vi "Autonomous Independent.vi"() -> ()   [LabVIEW 2014]
doc: "This VI is called when autonomous begins, and will automatically be terminated when autonomous ends. You can carry out timed or sensor driven robot movement independently without needing to return to the caller."
uses:
  Robot Global Data.vi
  <vilib>/Rock Robotics/WPI/RobotDrive/WPI_RobotDriveGetSetRefNum.vi
  <vilib>/Rock Robotics/WPI/RobotDrive/WPI_RobotDriveMecanumDrive_Cartesian.vi
panel:
  out "Current Movement, for debugging":T1 {"Z Joystick Value" scale=-1.0..1.0; "Y Joystick Value" scale=1.0..-1.0; "X Joystick Value" scale=-1.0..1.0}
  in  "Array of robot movements":T2(array[cluster]) {"Z Joystick Value" scale=-1.0..1.0; "Y Joystick Value" scale=1.0..-1.0; "X Joystick Value" scale=-1.0..1.0}
  # "Be sure to right-click and choose Data Operations>>Make Current Value default if you want to save the array values with the VI"
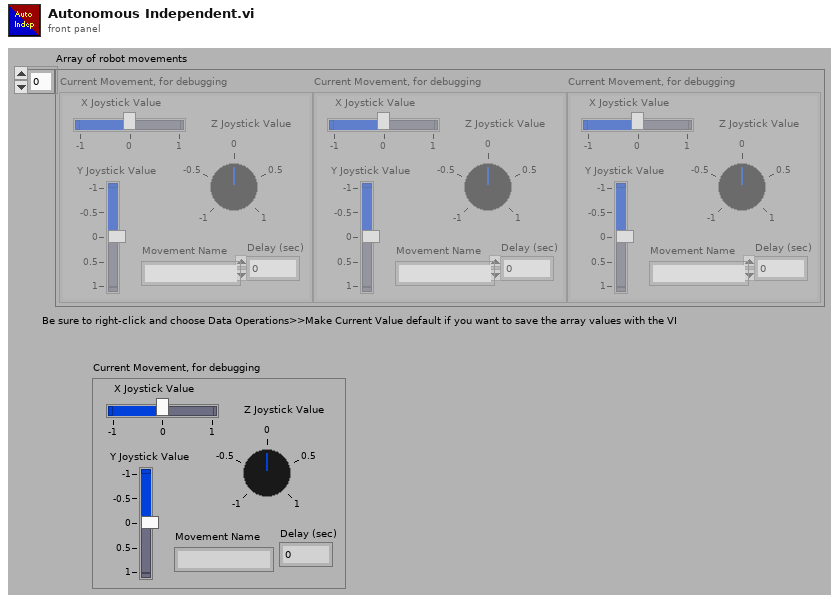
[diagram p1: front panel]
types:
  T1 = cluster{"X Joystick Value":dbl, "Y Joystick Value":dbl, "Z Joystick Value":dbl, "Delay (sec)":dbl, "Movement Name":string}
  T2 = cluster{"X Joystick Value":dbl, "Y Joystick Value":dbl, "Z Joystick Value":dbl, "Delay (sec)":dbl, "Movement Name":string}[]
  T3 = typedef "WPI_RobotDriveDevRef.ctl" = cluster{"DevStatus":errorcluster, "Motors[]":T4[], "Square Inputs":bool, "Max Output":dbl}
  T4 = typedef "WPI_MotorControlDeviceRef.ctl" = cluster{"DeviceStatus":errorcluster, "Type":enum16{"PWM", "CAN"}, "PWM":cluster{"Digital Module":T5, "PWM Channel":T6, "DeadBand":T7}, "CAN":cluster{"Device Number":u8, "Control Mode":T8, "Semaphore":T9, "Max Vout":dbl}, "Invert":bool, "TransformRef":T10, "InvTransformRef":T10}
  T5 = typedef "FPGA_TypedefDigitalModule.ctl" = enum16{"Digital Module 1", "Digital Module 2"}
  T6 = typedef "FPGA_DIOPWMChannel.ctl" = enum8{"PWM 1", "PWM 2", "PWM 3", "PWM 4", "PWM 5", "PWM 6", "PWM 7", "PWM 8", "PWM 9", "PWM 10", "Invalid"}
  T7 = typedef "WPI_PWMDeadband.ctl" = cluster{"Name":string, "maxPositivePwm":i32, "minPositivePwm":i32, "centerPwm":i32, "maxNegativePwm":i32, "minNegativePwm":i32, "angularRange":u16}
  T8 = typedef "WPI_CANJaguar_ControlMode.ctl" = enum8{"Percent VBus", "Current", "Speed", "Position", "Voltage"}
  T9 = typedef "Semaphore RefNum" = refnum<k1>
  T10 = typedef "WPI_PWMTransform_ConPane.ctl" = refnum<vi>
  T11 = typedef "WPI_DigitalInputDevRef.ctl" = cluster{"DevStatus":errorcluster, "DIO Channel":T12, "Digital Module":T5}
  T12 = typedef "FPGA_DIOChannel.ctl" = enum8{"DIO 1", "DIO 2", "DIO 3", "DIO 4", "DIO 5", "DIO 6", "DIO 7", "DIO 8", "DIO 9", "DIO 10", "DIO 11", "DIO 12", "DIO 13", "DIO 14", "Invalid"}
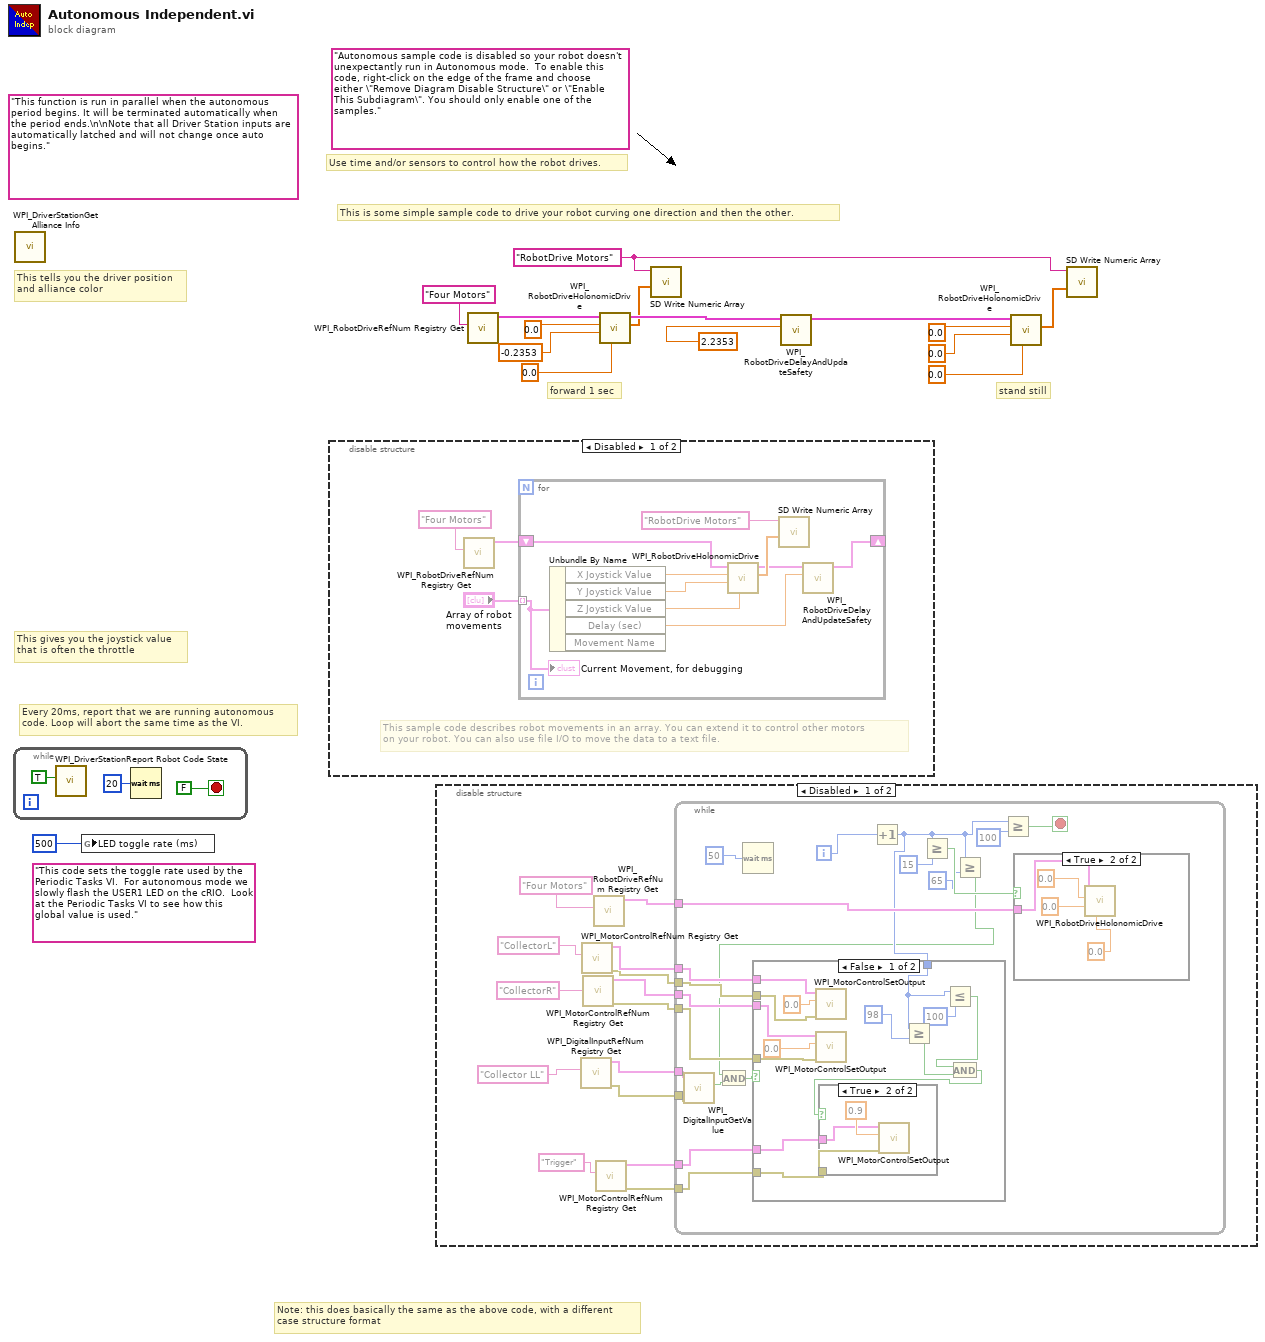
[diagram p0: block diagram]
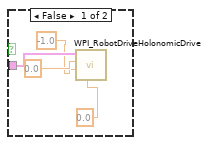
[diagram p2: hidden frame]
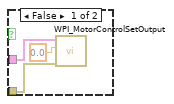
[diagram p3: hidden frame]
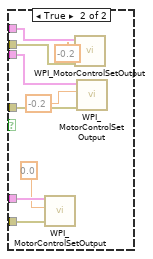
[diagram p4: hidden frame]
diagram:
  w4 = "RobotDrive Motors" ("Name")
  (unwired) "This code sets the toggle rate used by the Periodic Tasks VI.  For autonomous mode we slowly flash the USER1 LED on the cRIO.  Look at the Periodic Tasks VI to see how this global value is used."
  (unwired) "Autonomous sample code is disabled so your robot doesn't unexpectantly run in Autonomous mode.  To enable this code, right-click on the edge of the frame and choose either \"Remove Diagram Disable Structure\" or \"Enable This Subdiagram\". You should only enable one of the samples."
  (unwired) "This function is run in parallel when the autonomous period begins. It will be terminated automatically when the period ends.\n\nNote that all Driver Station inputs are automatically latched and will not change once auto begins."
  # "This is some simple sample code to drive your robot curving one direction and then the other."
  # "stand still"
  # "forward 1 sec"
  # "Note: this does basically the same as the above code, with a different\ncase structure format"
  # "Every 20ms, report that we are running autonomous\ncode. Loop will abort the same time as the VI."
  # "This gives you the joystick value\nthat is often the throttle"
  # "Use time and/or sensors to control how the robot drives."
  # "This tells you the driver position\nand alliance color"
  n1 = while {
    stop <- FALSE stop-if-true
    n2 = call <vilib>:"WPI_DriverStationReport Robot Code State.vi"("Autonomous"=TRUE) -> ()  [unwired: 10 in, 1 out]
    n3 = Wait (ms)(milliseconds to wait=u32 20) -> ()  [unwired: 1 out]
  }
  n4 = call <vilib>:"WPI_DriverStationGet Alliance Info.vi"() -> ()  [unwired: 12 out]
  n5 = global write "Robot Global Data.vi" "LED toggle rate (ms)"(u32 500 ("LED ms toggle rate")) -> ()
  n6 = disable-structure shown="Disabled" {
    frame Disabled {
      # "This sample code describes robot movements in an array. You can extend it to control other motors\non your robot. You can also use file I/O to move the data to a text file."
      n7 = call <vilib>:"WPI_RobotDriveRefNum Registry Get.vi"("refnum name"="Four Motors") -> ("RobotDriveDevRef"=w20:T3)  [unwired: 1 in, 9 out]
      n8 = for {
        shift-right: [w27] -> _
        shift-left: w20 -> [w28]
        tunnel: "Array of robot movements" -> [w23] mode=indexing
        n9 = Unbundle By Name(w23) -> ("X Joystick Value"=w26:dbl, "Y Joystick Value"=w25:dbl, "Z Joystick Value"=w22:dbl, "Delay (sec)"=w24:dbl)  [unwired: 1 out]
        n10 = call-poly <vilib>:"WPI_RobotDriveHolonomicDrive.vi"("Rotation"=w22, "Y"=w25, "X"=w26, "RobotDriveDevRef"=w28) -> ("Motor Values"=w30:dbl[], "RobotDriveDevRef"=w29:T3)  [unwired: 5 in, 1 out]
        n11 = call <vilib>:"SD Write Numeric Array.vi"("Numeric Array"=w30, "Name"="RobotDrive Motors") -> ()  [unwired: 8 in, 2 out]
        n12 = call <vilib>:"WPI_RobotDriveDelayAndUpdateSafety.vi"("Delay (s)"=w24, "RobotDriveDevRef"=w29) -> ("RobotDriveDevRef 2"=w27:T3)  [unwired: 8 in, 1 out]
        "Current Movement, for debugging" <- w23
      }
    }
    frame Enabled {
    }
  }
  n13 = disable-structure shown="Disabled" {
    frame Disabled {
      n14 = call <vilib>:"WPI_DigitalInputRefNum Registry Get.vi"("refnum name"="Collector LL") -> ("error out"=w32:errorcluster, "DigitalInputDevRef"=w33:T11)  [unwired: 9 in]
      n15 = call <vilib>:"WPI_MotorControlRefNum Registry Get.vi"("refnum name"="CollectorL") -> ("error out"=w38:errorcluster, "MotorControlDevRef"=w41:T4)  [unwired: 9 in]
      n16 = call <vilib>:"WPI_MotorControlRefNum Registry Get.vi"("refnum name"="CollectorR") -> ("error out"=w37:errorcluster, "MotorControlDevRef"=w42:T4)  [unwired: 9 in]
      n17 = call <vilib>:"WPI_RobotDriveRefNum Registry Get.vi"("refnum name"="Four Motors") -> ("RobotDriveDevRef"=w45:T3)  [unwired: 1 in, 9 out]
      n18 = call <vilib>:"WPI_MotorControlRefNum Registry Get.vi"("refnum name"="Trigger") -> ("error out"=w34:errorcluster, "MotorControlDevRef"=w35:T4)  [unwired: 9 in]
      n19 = while {
        tunnel: w45 -> [w56]
        tunnel: w42 -> [w61]
        tunnel: w41 -> [w62]
        tunnel: w38 -> [w60]
        tunnel: w37 -> [w59]
        tunnel: w35 -> [w55]
        tunnel: w34 -> [w54]
        tunnel: w33 -> [w53]
        tunnel: w32 -> [w52]
        i -> [w64]
        stop <- w57 stop-if-true
        n20 = call <vilib>:"WPI_DigitalInputGetValue.vi"("error in (no error)"=w52, "DigitalInputDevRef"=w53) -> ("Value"=w51:bool)  [unwired: 7 in, 2 out]
        n21 = Wait (ms)(milliseconds to wait=50) -> ()  [unwired: 1 out]
        n22 = Increment(x=w64) -> (x+1=w47:i32)
        n23 = Greater Or Equal?(x=w47, y=15) -> (x >= y?=w49:bool)
        n24 = Greater Or Equal?(x=w47, y=65) -> (x >= y?=w46:bool)
        n25 = And(x=w46, y=w51) -> (x .and. y?=w50:bool)
        n26 = case shown="False" w50 {
          tunnel: w62 -> [w85 w102]
          tunnel: w61 -> [w83 w101]
          tunnel: w60 -> [w84 w99]
          tunnel: w59 -> [w82 w100]
          tunnel: w55 -> [w80 w96]
          tunnel: w47 -> [w81 _]
          tunnel: w54 -> [w79 w95]
          frame False {
            n27 = call <vilib>:"WPI_MotorControlSetOutput.vi"("error in (no error)"=w84, "Output"=0.0, "MotorControlDevRef"=w85) -> ()  [unwired: 6 in, 3 out]
            n28 = call <vilib>:"WPI_MotorControlSetOutput.vi"("error in (no error)"=w82, "Output"=0.0, "MotorControlDevRef"=w83) -> ()  [unwired: 6 in, 3 out]
            n29 = Greater Or Equal?(x=w81, y=98) -> (x >= y?=w75:bool)
            n30 = Less Or Equal?(x=w81, y=100) -> (x <= y?=w76:bool)
            n31 = And(x=w76, y=w75) -> (x .and. y?=w74:bool)
            n32 = case shown="True" w74 {
              tunnel: w80 -> [w89 w91]
              tunnel: w79 -> [w90 w93]
              frame False {
                n33 = call <vilib>:"WPI_MotorControlSetOutput.vi"("error in (no error)"=w90, "Output"=0.0, "MotorControlDevRef"=w89) -> ()  [unwired: 6 in, 3 out]
              }
              frame True {
                n34 = call <vilib>:"WPI_MotorControlSetOutput.vi"("error in (no error)"=w93, "Output"=0.9, "MotorControlDevRef"=w91) -> ()  [unwired: 6 in, 3 out]
              }
            }
          }
          frame True {
            n35 = call <vilib>:"WPI_MotorControlSetOutput.vi"("error in (no error)"=w95, "Output"=0.0, "MotorControlDevRef"=w96) -> ()  [unwired: 6 in, 3 out]
            n36 = call <vilib>:"WPI_MotorControlSetOutput.vi"("error in (no error)"=w99, "Output"=-0.2, "MotorControlDevRef"=w102) -> ()  [unwired: 6 in, 3 out]
            n37 = call <vilib>:"WPI_MotorControlSetOutput.vi"("error in (no error)"=w100, "Output"=-0.2, "MotorControlDevRef"=w101) -> ()  [unwired: 6 in, 3 out]
          }
        }
        n38 = Greater Or Equal?(x=w47, y=100) -> (x >= y?=w57:bool)
        n39 = case shown="True" w49 {
          tunnel: w56 -> [w69 w70]
          frame False {
            n40 = call-poly <vilib>:"WPI_RobotDriveHolonomicDrive.vi"("Rotation"=0.0, "Y"=-1.0, "X"=0.0, "RobotDriveDevRef"=w69) -> ()  [unwired: 5 in, 3 out]
          }
          frame True {
            n41 = call-poly <vilib>:"WPI_RobotDriveHolonomicDrive.vi"("Rotation"=0.0, "Y"=0.0, "X"=0.0, "RobotDriveDevRef"=w70) -> ()  [unwired: 5 in, 3 out]
          }
        }
      }
    }
    frame Enabled {
    }
  }
  n42 = call <vilib>:"WPI_RobotDriveRefNum Registry Get.vi"("refnum name"="Four Motors") -> ("RobotDriveDevRef"=w7:T3)  [unwired: 1 in, 9 out]
  n43 = call-poly <vilib>:"WPI_RobotDriveHolonomicDrive.vi"("Rotation"=0.0, "Y"=-0.2353 ("X axis value"), "X"=0.0 ("X axis value"), "RobotDriveDevRef"=w7) -> ("Motor Values"=w6:dbl[], "RobotDriveDevRef"=w10:T3)  [unwired: 5 in, 1 out]
  n44 = call <vilib>:"SD Write Numeric Array.vi"("Numeric Array"=w6, "Name"=w4) -> ()  [unwired: 8 in, 2 out]
  n45 = call <vilib>:"WPI_RobotDriveDelayAndUpdateSafety.vi"("Delay (s)"=2.2353, "RobotDriveDevRef"=w10) -> ("RobotDriveDevRef 2"=w1:T3)  [unwired: 8 in, 1 out]
  n46 = call-poly <vilib>:"WPI_RobotDriveHolonomicDrive.vi"("Rotation"=0.0 ("X axis value"), "Y"=0.0 ("X axis value"), "X"=0.0 ("X axis value"), "RobotDriveDevRef"=w1) -> ("Motor Values"=w5:dbl[])  [unwired: 5 in, 2 out]
  n47 = call <vilib>:"SD Write Numeric Array.vi"("Numeric Array"=w5, "Name"=w4) -> ()  [unwired: 8 in, 2 out]
